vi "GA_Adjust Mutation Rate.vi"(8 "Parameters in":T1={"Population size"=0, "Generations no."=0, "Crossover probabality"=0.0, "Mutation mode"=enum."one-point, fixed rate", "Creep mutation"=FALSE, "Mutation rate"=0.005, "Min mutation rate"=0.0, "Max mutation rate"=0.0, "Relative fitness differential"=0.0, "Reproduction plan"=enum."Full generational replacement", "Elitism"=FALSE, "FeaturesPerChannel"=0} {"Relative fitness differential" min=0.0 max=1.0; "Max mutation rate" min=0.0 max=1.0; "Min mutation rate" min=0.0 max=1.0; "Mutation rate" min=0.0 max=1.0; "Crossover probabality" min=0.0 max=1.0; "Generations no." min=1; "Population size" min=1}, 11 "Population":T2) -> (0 "Parameters out":T1={"Population size"=0, "Generations no."=0, "Crossover probabality"=0.0, "Mutation mode"=enum."one-point, fixed rate", "Creep mutation"=FALSE, "Mutation rate"=0.005, "Min mutation rate"=0.0, "Max mutation rate"=0.0, "Relative fitness differential"=0.0, "Reproduction plan"=enum."Full generational replacement", "Elitism"=FALSE, "FeaturesPerChannel"=0} {"Relative fitness differential" min=0.0 max=1.0; "Max mutation rate" min=0.0 max=1.0; "Min mutation rate" min=0.0 max=1.0; "Mutation rate" min=0.0 max=1.0; "Crossover probabality" min=0.0 max=1.0; "Generations no." min=1; "Population size" min=1})   [LabVIEW 2016, in "GA.lvlib"]
doc: "Adjusts mutation rate according to status of the population and parameters - speeds up mutation for low population spread and slows down for high."
uses:
  GA.lvlib
  GA_tPopulation.ctl
  GA_tParameters.ctl
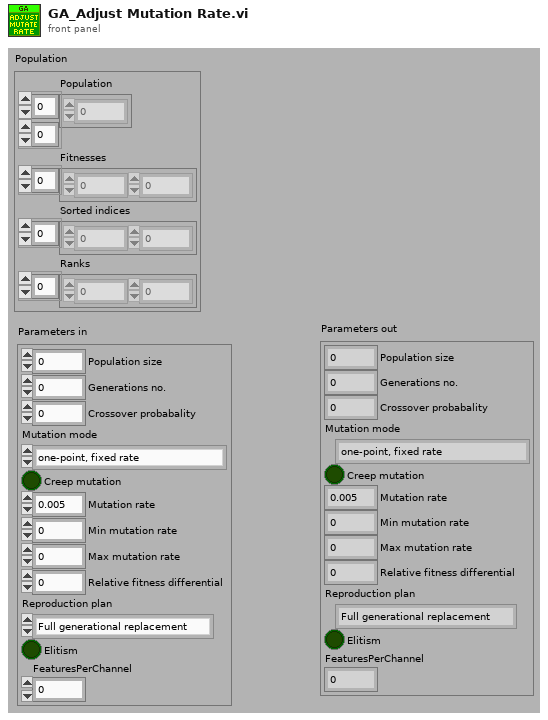
[diagram p1: front panel]
types:
  T1 = typedef "GA.lvlib/GA_tParameters.ctl" = cluster{"Population size":i32, "Generations no.":i32, "Crossover probabality":dbl, "Mutation mode":enum16{"one-point, fixed rate", "one-point, fitness-adjustable rate", "one-point, distance-adjustable rate"}, "Creep mutation":bool, "Mutation rate":dbl, "Min mutation rate":dbl, "Max mutation rate":dbl, "Relative fitness differential":dbl, "Reproduction plan":enum16{"Full generational replacement", "Steady-state-replace-random", "Steady-state-replace-worst"}, "Elitism":bool, "FeaturesPerChannel":i32}
  T2 = typedef "GA.lvlib/GA_tPopulation.ctl" = cluster{"Population":i8[][], "Fitnesses":dbl[], "Sorted indices":i32[], "Ranks":i32[]}
  T3 = enum16{"one-point, fixed rate", "one-point, fitness-adjustable rate", "one-point, distance-adjustable rate"}
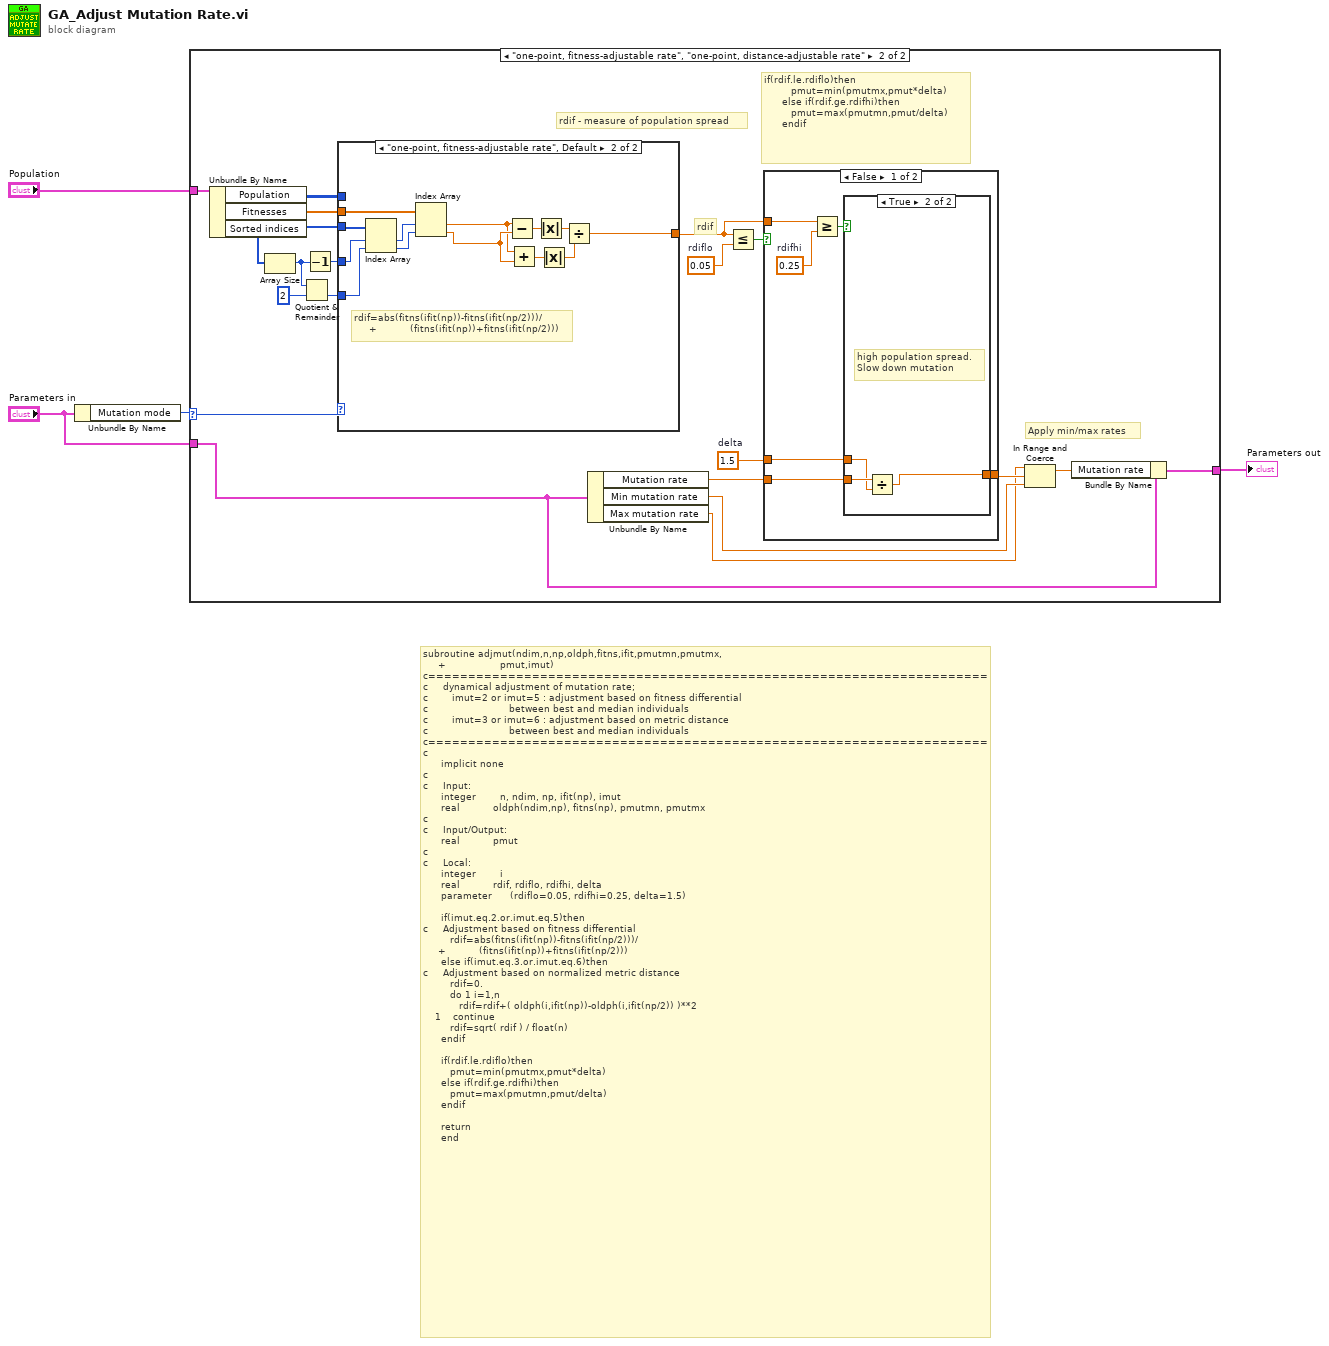
[diagram p0: block diagram]
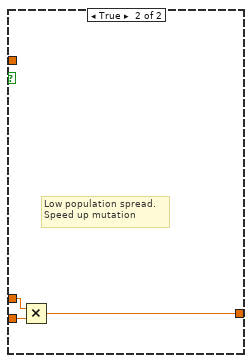
[diagram p4: hidden frame]
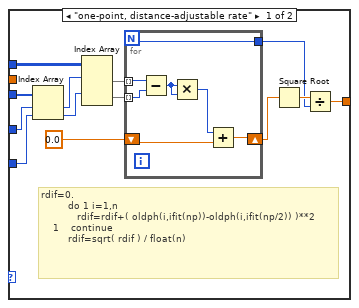
[diagram p5: hidden frame]
diagram:
  # "subroutine adjmut(ndim,n,np,oldph,fitns,ifit,pmutmn,pmutmx,\n     +                  pmut,imut)\nc======================================================================\nc     dynamical adjustment of mutation rate;\nc        imut=2 or imut=5 : adjustment based on fitness differential\nc                           between best and median individuals\nc        imut=3 or imut=6 : adjustment based on metric distance\nc                           between best and median individuals\nc======================================================================\nc\n      implicit none\nc\nc     Input:\n      integer        n, ndim, np, ifit(np), imut\n      real           oldph(ndim,np), fitns(np), pmutmn, pmutmx\nc\nc     Input/Output:\n      real           pmut\nc\nc     Local:\n      integer        i\n      real           rdif, rdiflo, rdifhi, delta\n      parameter      (rdiflo=0.05, rdifhi=0.25, delta=1.5)\n\n      if(imut.eq.2.or.imut.eq.5)then\nc     Adjustment based on fitness differential \n         rdif=abs(fitns(ifit(np))-fitns(ifit(np/2)))/\n     +           (fitns(ifit(np))+fitns(ifit(np/2)))\n      else if(imut.eq.3.or.imut.eq.6)then\nc     Adjustment based on normalized metric distance\n         rdif=0.\n         do 1 i=1,n\n            rdif=rdif+( oldph(i,ifit(np))-oldph(i,ifit(np/2)) )**2\n    1    continue\n         rdif=sqrt( rdif ) / float(n)\n      endif\n\n      if(rdif.le.rdiflo)then\n         pmut=min(pmutmx,pmut*delta)\n      else if(rdif.ge.rdifhi)then\n         pmut=max(pmutmn,pmut/delta)\n      endif\n \n      return\n      end"
  n1 = Unbundle By Name("Parameters in") -> ("Mutation mode"=w4:T3)
  n2 = case shown="\"one-point, fitness-adjustable rate\", \"one-point, distance-adjustable rate\"" w4 {
    selector: w4 -> [_ w25]
    tunnel: "Population" -> [_ w24]
    tunnel: "Parameters in" -> [w5 w8]
    tunnel: [w5 w6] -> w1
    frame "one-point, fixed rate", Default {
      # "Constant mutation rate"
    }
    frame "one-point, fitness-adjustable rate", "one-point, distance-adjustable rate" {
      w13 = 1.5  # delta
      w16 = 0.05  # rdiflo
      # "Apply min/max rates"
      # "rdif - measure of population spread"
      # "if(rdif.le.rdiflo)then\n         pmut=min(pmutmx,pmut*delta)\n      else if(rdif.ge.rdifhi)then\n         pmut=max(pmutmn,pmut/delta)\n      endif"
      # "rdif"
      n3 = Unbundle By Name(w24) -> ("Population"=w17:i8[][], "Fitnesses"=w21:dbl[], "Sorted indices"=w22:i32[])
      n4 = Array Size(array=w22) -> (size(s)=w20:i32)
      n5 = Quotient & Remainder(x=w20, y=2) -> (floor(x/y)=w18:i32)  [unwired: 1 out]
      n6 = Decrement(x=w20) -> (x-1=w23:i32)
      n7 = case shown="\"one-point, fitness-adjustable rate\", Default" w25 {
        tunnel: w23 -> [w50 w70]
        tunnel: w22 -> [w51 w71]
        tunnel: w21 -> [_ w69]
        tunnel: w18 -> [w49 w67]
        tunnel: [w44 w65] -> w12
        tunnel: w17 -> [w43 _]
        frame "one-point, distance-adjustable rate" {
          # "rdif=0.\n         do 1 i=1,n\n            rdif=rdif+( oldph(i,ifit(np))-oldph(i,ifit(np/2)) )**2\n    1    continue\n         rdif=sqrt( rdif ) / float(n)"
          n8 = Index Array(array=w51, index #1=w50, index #2=w49) -> (element #1=w42:i32, element #2=w41:i32)
          n9 = Index Array(array=w43, index (row) #1=w42, index (row) #2=w41) -> (element #1=w40:i8[], element #2=w39:i8[])  [unwired: 2 in]
          n10 = for {
            N -> [w54]
            shift-right: [w57] -> w47
            shift-left: 0.0 ("y") -> [w56]
            tunnel: [w54] -> w45
            tunnel: w40 -> [w53] mode=indexing
            tunnel: w39 -> [w52] mode=indexing
            n11 = Subtract(x=w53, y=w52) -> (x-y=w58:i8)
            n12 = Multiply(x=w58, y=w58) -> (x*y=w55:i8)
            n13 = Add(x=w55, y=w56) -> (x+y=w57:dbl)
          }
          n14 = Square Root(x=w47) -> (sqrt(x)=w46:dbl)
          n15 = Divide(x=w46, y=w45) -> (x/y=w44:dbl)
        }
        frame "one-point, fitness-adjustable rate", Default {
          # "rdif=abs(fitns(ifit(np))-fitns(ifit(np/2)))/\n     +           (fitns(ifit(np))+fitns(ifit(np/2)))"
          n16 = Index Array(array=w71, index #1=w70, index #2=w67) -> (element #1=w68:i32, element #2=w66:i32)
          n17 = Index Array(array=w69, index #1=w68, index #2=w66) -> (element #1=w61:dbl, element #2=w64:dbl)
          n18 = Subtract(x=w61, y=w64) -> (x-y=w63:dbl)
          n19 = Add(x=w61, y=w64) -> (x+y=w60:dbl)
          n20 = Absolute Value(x=w63) -> (abs(x)=w62:dbl)
          n21 = Absolute Value(x=w60) -> (abs(x)=w59:dbl)
          n22 = Divide(x=w62, y=w59) -> (x/y=w65:dbl)
        }
      }
      n23 = Unbundle By Name(w8) -> ("Mutation rate"=w14:dbl, "Min mutation rate"=w10:dbl, "Max mutation rate"=w9:dbl)
      n24 = Less Or Equal?(x=w12, y=w16) -> (x <= y?=w15:bool)
      n25 = case shown="False" w15 {
        tunnel: w14 -> [w27 w38]
        tunnel: w13 -> [w28 w37]
        tunnel: [w26 w36] -> w11
        tunnel: w12 -> [w31 _]
        frame False {
          w30 = 0.25  # rdifhi
          n26 = Greater Or Equal?(x=w31, y=w30) -> (x >= y?=w29:bool)
          n27 = case shown="True" w29 {
            tunnel: w28 -> [_ w34]
            tunnel: w27 -> [w32 w35]
            tunnel: [w32 w33] -> w26
            frame False {
            }
            frame True {
              # "high population spread.\nSlow down mutation"
              n28 = Divide(x=w35, y=w34) -> (x/y=w33:dbl)
            }
          }
        }
        frame True {
          # "Low population spread.\nSpeed up mutation"
          n29 = Multiply(x=w37, y=w38) -> (x*y=w36:dbl)
        }
      }
      n30 = In Range and Coerce(upper limit=w9, x=w11, lower limit=w10) -> (coerced(x)=w7:dbl)  [unwired: 1 out]
      n31 = Bundle By Name(cluster=w8, "Mutation rate"=w7) -> (w6:T1)
    }
  }
  "Parameters out" <- w1
